vi "Periodic Tasks.vi"(8 "error in":errorcluster) -> ()   [LabVIEW 2018]
doc: "This VI runs in parallel to other tasks. It can contain as many user-defined periodic loops as you need. These can carry out PID or other sorts of timed response."
uses:
  <vilib>/Rock Robotics/WPI/Utilities/WPI_GetSetVariantRefNum.vi
  Robot Global Data.vi
  <vilib>/Rock Robotics/Network Tables/NT Write Boolean.vi
  <vilib>/Rock Robotics/Network Tables/NT Write Number.vi
panel:
  out "Motor Speed Graph":dbl(graph)
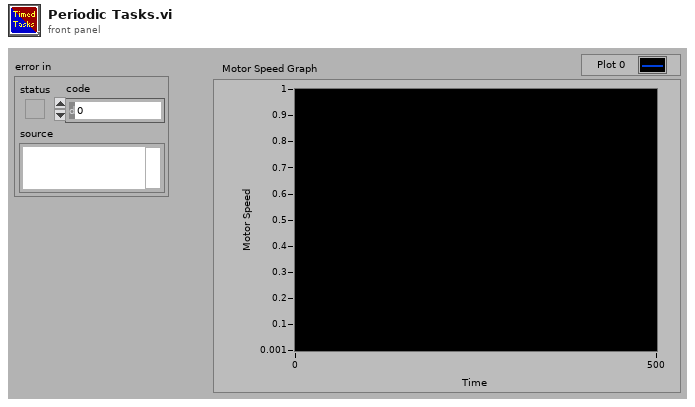
[diagram p1: front panel]
types:
  T1 = typedef "WPI_JoystickDevRef.ctl" = cluster{"Device":T2}
  T2 = typedef "WPI_JoystickDeviceEnum.ctl" = enum16{"USB 0", "USB 1", "USB 2", "USB 3", "USB 4", "USB 5"}
  T3 = cluster{"JoystickDevRef":T1, "JoystickDevRef":T1, "JoystickDevRef":T1}
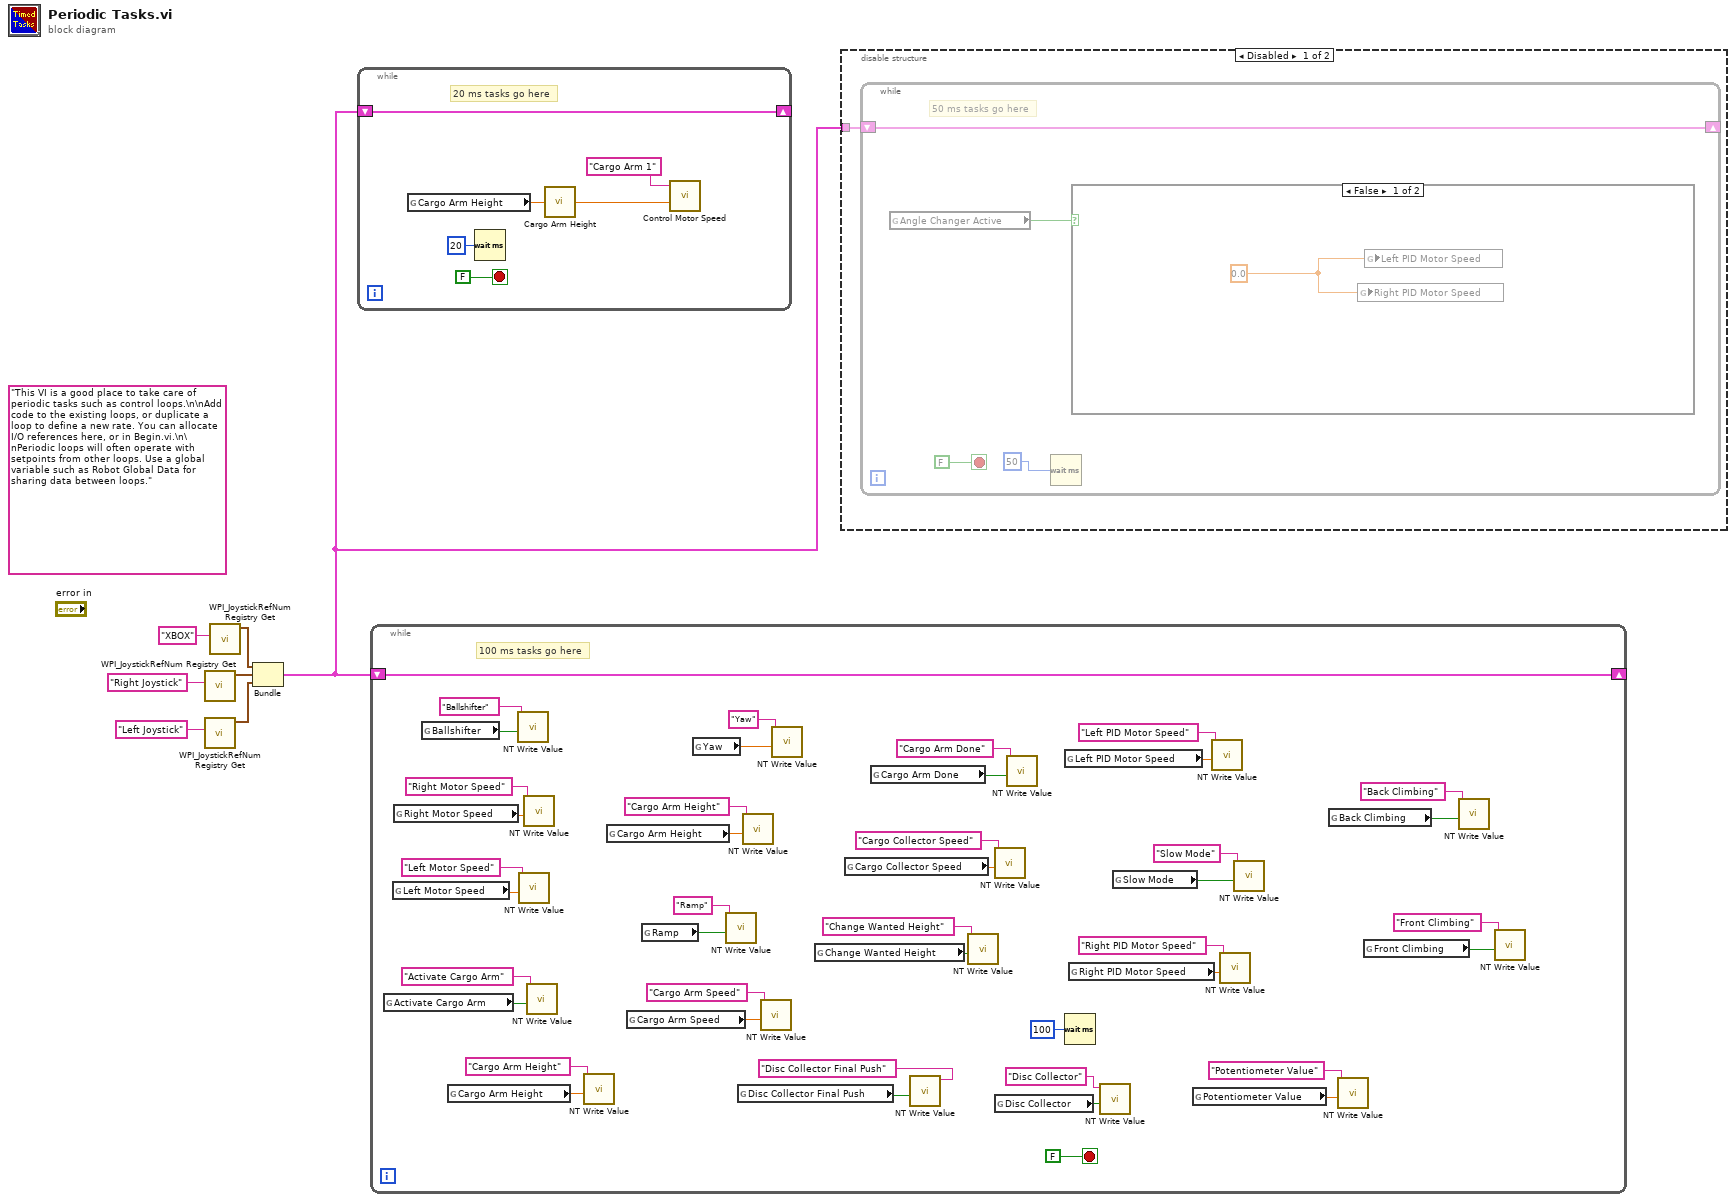
[diagram p0: block diagram]
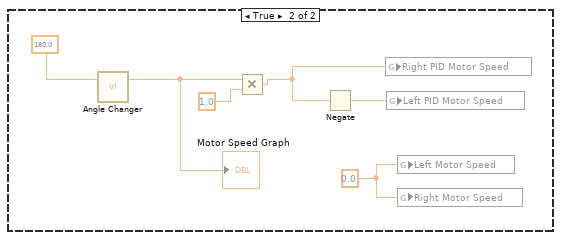
[diagram p2: hidden frame]
diagram:
  (unwired) "This VI is a good place to take care of periodic tasks such as control loops.\n\nAdd code to the existing loops, or duplicate a loop to define a new rate. You can allocate I/O references here, or in Begin.vi.\n\nPeriodic loops will often operate with setpoints from other loops. Use a global variable such as Robot Global Data for sharing data between loops."
  n1 = call <vilib>:"WPI_JoystickRefNum Registry Get.vi"("refnum name"="Right Joystick") -> ("JoystickDevRef"=w3:T1)  [unwired: 1 in, 9 out]
  n2 = call <vilib>:"WPI_JoystickRefNum Registry Get.vi"("refnum name"="Left Joystick") -> ("JoystickDevRef"=w2:T1)  [unwired: 1 in, 9 out]
  n3 = call <vilib>:"WPI_JoystickRefNum Registry Get.vi"("refnum name"="XBOX") -> ("JoystickDevRef"=w6:T1)  [unwired: 1 in, 9 out]
  n4 = Bundle("JoystickDevRef"=w6, "JoystickDevRef"=w3, "JoystickDevRef"=w2) -> (w1:T3)  [unwired: 1 out]
  n5 = while {
    shift-right: [w11] -> _
    shift-left: w1 -> [w11]
    stop <- FALSE stop-if-true
    # "20 ms tasks go here"
    n6 = global read "Robot Global Data.vi" "Cargo Arm Height"() -> (w10:dbl)
    n7 = Wait (ms)(milliseconds to wait=u32 20) -> ()  [unwired: 1 out]
    n8 = call "Cargo Arm Height.vi"("Wanted Distance"=w10) -> ("Arm Final Speed"=w8:dbl)
    n9 = call "Control Motor Speed.vi"("Speed"=w8, "Motor Name"="Cargo Arm 1") -> ()  [unwired: 2 in]
  }
  n10 = while {
    shift-right: [w54] -> _
    shift-left: w1 -> [w54]
    stop <- FALSE stop-if-true
    # "100 ms tasks go here"
    n11 = global read "Robot Global Data.vi" "Activate Cargo Arm"() -> (w42:bool)
    n12 = global read "Robot Global Data.vi" "Left Motor Speed"() -> (w51:dbl)
    n13 = global read "Robot Global Data.vi" "Right Motor Speed"() -> (w49:dbl)
    n14 = global read "Robot Global Data.vi" "Ballshifter"() -> (w53:bool)
    n15 = global read "Robot Global Data.vi" "Cargo Arm Height"() -> (w32:dbl)
    n16 = call-poly <vilib>:"NT Write Value.vi"("Boolean"=w53, "Name"="Ballshifter") -> ()  [unwired: 9 in, 1 out]
    n17 = call-poly <vilib>:"NT Write Value.vi"("Numeric"=w51, "Name"="Left Motor Speed") -> ()  [unwired: 9 in, 1 out]
    n18 = call-poly <vilib>:"NT Write Value.vi"("Numeric"=w49, "Name"="Right Motor Speed") -> ()  [unwired: 9 in, 1 out]
    n19 = call-poly <vilib>:"NT Write Value.vi"("Boolean"=w42, "Name"="Activate Cargo Arm") -> ()  [unwired: 9 in, 1 out]
    n20 = call-poly <vilib>:"NT Write Value.vi"("Numeric"=w32, "Name"="Cargo Arm Height") -> ()  [unwired: 9 in, 1 out]
    n21 = global read "Robot Global Data.vi" "Cargo Arm Height"() -> (w20:dbl)
    n22 = global read "Robot Global Data.vi" "Cargo Arm Speed"() -> (w40:dbl)
    n23 = global read "Robot Global Data.vi" "Ramp"() -> (w44:bool)
    n24 = global read "Robot Global Data.vi" "Yaw"() -> (w46:dbl)
    n25 = call-poly <vilib>:"NT Write Value.vi"("Boolean"=w44, "Name"="Ramp") -> ()  [unwired: 9 in, 1 out]
    n26 = global read "Robot Global Data.vi" "Disc Collector Final Push"() -> (w29:bool)
    n27 = call-poly <vilib>:"NT Write Value.vi"("Numeric"=w20, "Name"="Cargo Arm Height") -> ()  [unwired: 9 in, 1 out]
    n28 = call-poly <vilib>:"NT Write Value.vi"("Numeric"=w40, "Name"="Cargo Arm Speed") -> ()  [unwired: 9 in, 1 out]
    n29 = call-poly <vilib>:"NT Write Value.vi"("Numeric"=w46, "Name"="Yaw") -> ()  [unwired: 9 in, 1 out]
    n30 = global read "Robot Global Data.vi" "Change Wanted Height"() -> (w34:bool)
    n31 = global read "Robot Global Data.vi" "Cargo Collector Speed"() -> (w38:dbl)
    n32 = global read "Robot Global Data.vi" "Cargo Arm Done"() -> (w36:bool)
    n33 = call-poly <vilib>:"NT Write Value.vi"("Boolean"=w29, "Name"="Disc Collector Final Push") -> ()  [unwired: 9 in, 1 out]
    n34 = call-poly <vilib>:"NT Write Value.vi"("Boolean"=w34, "Name"="Change Wanted Height") -> ()  [unwired: 9 in, 1 out]
    n35 = call-poly <vilib>:"NT Write Value.vi"("Numeric"=w38, "Name"="Cargo Collector Speed") -> ()  [unwired: 9 in, 1 out]
    n36 = global read "Robot Global Data.vi" "Disc Collector"() -> (w31:bool)
    n37 = call-poly <vilib>:"NT Write Value.vi"("Boolean"=w36, "Name"="Cargo Arm Done") -> ()  [unwired: 9 in, 1 out]
    n38 = global read "Robot Global Data.vi" "Left PID Motor Speed"() -> (w24:dbl)
    n39 = Wait (ms)(milliseconds to wait=u32 100) -> ()  [unwired: 1 out]
    n40 = global read "Robot Global Data.vi" "Right PID Motor Speed"() -> (w22:dbl)
    n41 = call-poly <vilib>:"NT Write Value.vi"("Boolean"=w31, "Name"="Disc Collector") -> ()  [unwired: 9 in, 1 out]
    n42 = global read "Robot Global Data.vi" "Slow Mode"() -> (w26:bool)
    n43 = global read "Robot Global Data.vi" "Potentiometer Value"() -> (w18:dbl)
    n44 = call-poly <vilib>:"NT Write Value.vi"("Numeric"=w24, "Name"="Left PID Motor Speed") -> ()  [unwired: 9 in, 1 out]
    n45 = call-poly <vilib>:"NT Write Value.vi"("Numeric"=w22, "Name"="Right PID Motor Speed") -> ()  [unwired: 9 in, 1 out]
    n46 = call-poly <vilib>:"NT Write Value.vi"("Boolean"=w26, "Name"="Slow Mode") -> ()  [unwired: 9 in, 1 out]
    n47 = global read "Robot Global Data.vi" "Back Climbing"() -> (w16:bool)
    n48 = call-poly <vilib>:"NT Write Value.vi"("Numeric"=w18, "Name"="Potentiometer Value") -> ()  [unwired: 9 in, 1 out]
    n49 = global read "Robot Global Data.vi" "Front Climbing"() -> (w14:bool)
    n50 = call-poly <vilib>:"NT Write Value.vi"("Boolean"=w16, "Name"="Back Climbing") -> ()  [unwired: 9 in, 1 out]
    n51 = call-poly <vilib>:"NT Write Value.vi"("Boolean"=w14, "Name"="Front Climbing") -> ()  [unwired: 9 in, 1 out]
  }
  n52 = disable-structure shown="Disabled" {
    disable-tunnel: w1 -> [w57 _]
    frame Disabled {
      n53 = while {
        shift-right: [w59] -> _
        shift-left: w57 -> [w59]
        stop <- FALSE stop-if-true
        # "50 ms tasks go here"
        n54 = global read "Robot Global Data.vi" "Angle Changer Active"() -> (w58:bool)
        n55 = Wait (ms)(milliseconds to wait=u32 50) -> ()  [unwired: 1 out]
        n56 = case shown="False" w58 {
          frame False {
            w62 = 0.0 ("Left PID Motor Speed")
            n57 = global write "Robot Global Data.vi" "Right PID Motor Speed"(w62) -> ()
            n58 = global write "Robot Global Data.vi" "Left PID Motor Speed"(w62) -> ()
          }
          frame True {
            w63 = 0.0
            n59 = call "Angle Changer.vi"("Angle"=180.0) -> ("Output"=w66:dbl)  [unwired: 1 in, 1 out]
            "Motor Speed Graph" <- w66
            n60 = Multiply(x=w66, y=1.0) -> (x*y=w65:dbl)
            n61 = Negate(x=w65) -> (-x=w68:dbl)
            n62 = global write "Robot Global Data.vi" "Right PID Motor Speed"(w65) -> ()
            n63 = global write "Robot Global Data.vi" "Left PID Motor Speed"(w68) -> ()
            n64 = global write "Robot Global Data.vi" "Left Motor Speed"(w63) -> ()
            n65 = global write "Robot Global Data.vi" "Right Motor Speed"(w63) -> ()
          }
        }
      }
    }
    frame Enabled {
    }
  }
